vi "Error Handler Terminate.vi"(8 "error in (no error)":errorcluster) -> (0 "error out":errorcluster)   [LabVIEW 2011]
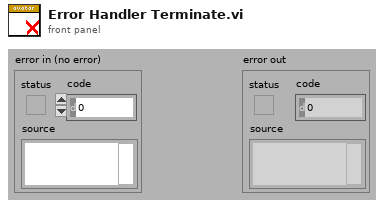
[diagram p1: front panel]
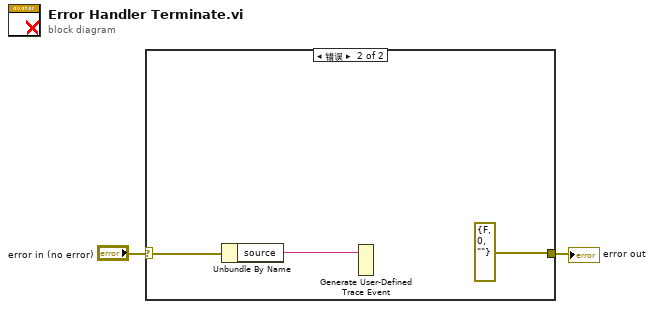
[diagram p0: block diagram]
diagram:
  n1 = case shown="错误" "error in (no error)" {
    selector: "error in (no error)" -> [w3 w4]
    tunnel: [w3 errorcluster {"status"=FALSE, "code"=0, "source"=""} ("error IO")] -> w2
    frame No Error {
    }
    frame Error {
      n2 = Unbundle By Name(w4) -> ("source"=w5:string)
      n3 = Generate User-Defined Trace Event(2:w5) -> ()  [unwired: 1 in]
    }
  }
  "error out" <- w2
